vi "HardwareRead.vi"(8 "Error In":errorcluster, 10 "Setup":T2={"DUT"={"Count"=1, "Wirings"=[], "Names"=[]}, "Log"={"Start"={"Trigger Type"=enum."Immediate", "Timer (sec)"=0.0, "Digital IO Line"=0, "Digital IO Edge"=enum."Rising"}, "Rollover"={"Trigger Type"=enum."None", "Timer (sec)"=0.0, "File Size (MB)"=0, "Digital IO Line"=0, "Digital IO Edge"=enum."Rising"}, "Stop"={"Trigger Type"=enum."None", "Timer (sec)"=0.0, "File Size (MB)"=0, "Digital IO Line"=0, "Digital IO Edge"=enum."Rising"}}, "Trigger"={"Input"={"Type"=enum."None", "Timeout (ms)"=0, "Delay (ms)"=0, "Digital IO Line (1-14)"=0, "Digital IO Mode"=enum."Falling"}, "Output"={"Type"=enum."None", "Delay (ms)"=0, "Digital IO Line (1-14)"=0, "Digital IO Mode"=enum."Falling", "Digital IO Pulse Width (sec)"=0.0}}, "Sources"=[], "Measures"=[]} {"Measures"."Count" min=1 step=1; "Trigger"."Output"."Digital IO Line (1-14)" min=1 max=14 step=1}, 11 "Keithley 2602 In":refnum<visa-resource-name>) -> (0 "Error Out":errorcluster, 2 "Hardware Display Data":T1, 3 "Keithley 2602 Out":refnum<visa-resource-name>)   [LabVIEW 2013]
uses:
  Setup.ctl
  DUTConfiguration.ctl
  driver/Public/Controls/SMUSense.ctl
  LogConfiguration.ctl
  LogStartConfiguration.ctl
  LogStartTriggerType.ctl
  LogDigitalIOTriggerEdge.ctl
  LogRolloverConfiguration.ctl
  LogRolloverTriggerType.ctl
  LogStopConfiguration.ctl
  LogStopTriggerType.ctl
  TriggerConfiguration.ctl
  TriggerInputConfiguration.ctl
  TriggerInputType.ctl
  driver/Public/Controls/TriggerMode.ctl
  TriggerOutputConfiguration.ctl
  TriggerOutputType.ctl
  SourceConfiguration.ctl
  SourceFunction.ctl
  MeasureConfiguration.ctl
  HardwareDisplayData.ctl
  HardwareAbortGlobalAction.ctl
  driver/Keithley-2602.lvlib
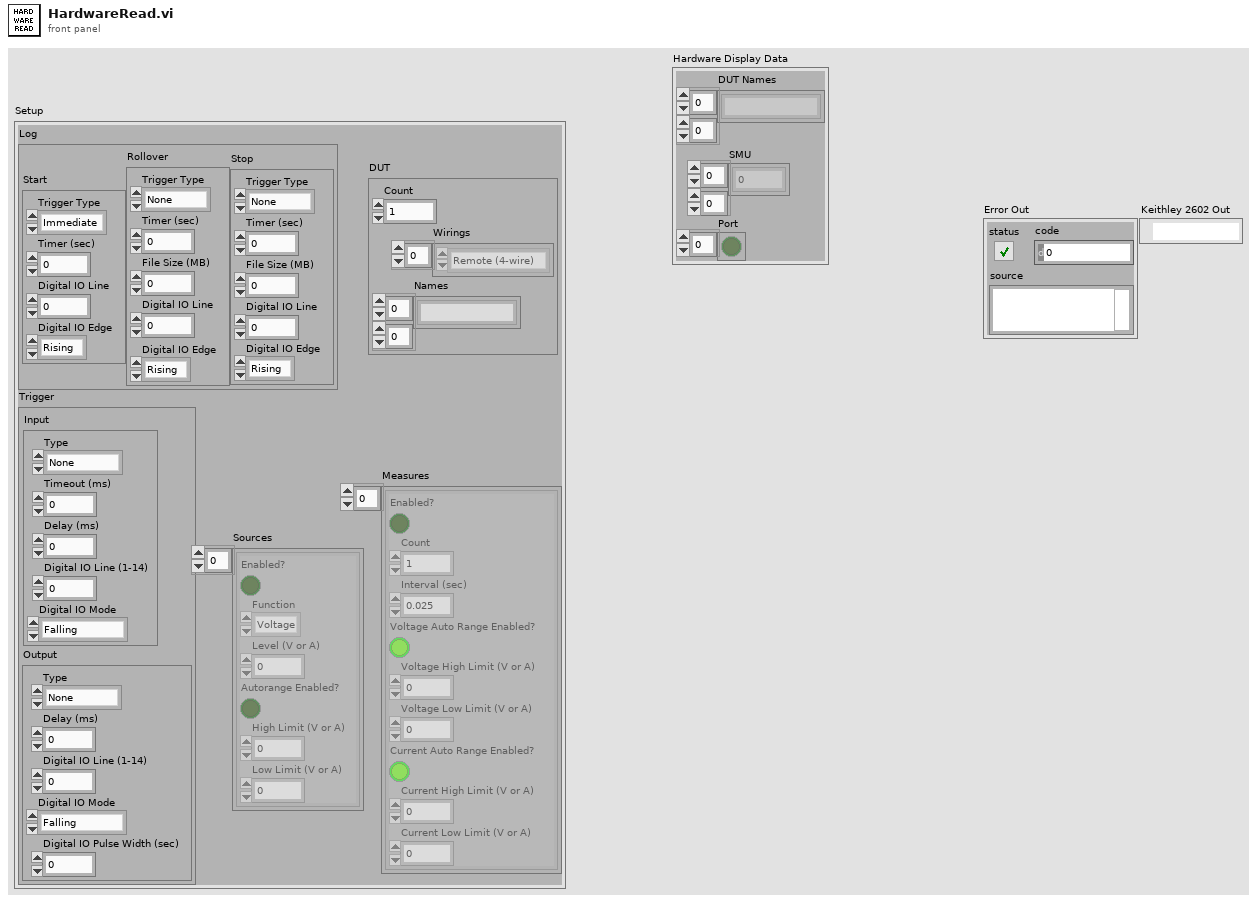
[diagram p1: front panel]
types:
  T1 = typedef "HardwareDisplayData.ctl" = cluster{"DUT Names":string[][], "SMU":dbl[][], "Port":bool[]}
  T2 = typedef "Setup.ctl" = cluster{"DUT":T3, "Log":T5, "Trigger":T13, "Sources":T19[], "Measures":T21[]}
  T3 = typedef "DUTConfiguration.ctl" = cluster{"Count":u32, "Wirings":T4[], "Names":string[][]}
  T4 = typedef "Keithley-2602.lvlib/SMUSense.ctl" = enum16{"Local (2-wire)", "Remote (4-wire)", "Calibration"}
  T5 = typedef "LogConfiguration.ctl" = cluster{"Start":T6, "Rollover":T9, "Stop":T11}
  T6 = typedef "LogStartConfiguration.ctl" = cluster{"Trigger Type":T7, "Timer (sec)":dbl, "Digital IO Line":u8, "Digital IO Edge":T8}
  T7 = typedef "LogStartTriggerType.ctl" = enum16{"Immediate", "User", "Timer", "Digital IO"}
  T8 = typedef "LogDigitalIOTriggerEdge.ctl" = enum16{"Rising", "Falling"}
  T9 = typedef "LogRolloverConfiguration.ctl" = cluster{"Trigger Type":T10, "Timer (sec)":dbl, "File Size (MB)":u32, "Digital IO Line":u8, "Digital IO Edge":T8}
  T10 = typedef "LogRolloverTriggerType.ctl" = enum16{"None", "Timer", "File Size", "Digital IO"}
  T11 = typedef "LogStopConfiguration.ctl" = cluster{"Trigger Type":T12, "Timer (sec)":dbl, "File Size (MB)":u32, "Digital IO Line":u8, "Digital IO Edge":T8}
  T12 = typedef "LogStopTriggerType.ctl" = enum16{"None", "User", "Timer", "File Size", "Digital IO"}
  T13 = typedef "TriggerConfiguration.ctl" = cluster{"Input":T14, "Output":T17}
  T14 = typedef "TriggerInputConfiguration.ctl" = cluster{"Type":T15, "Timeout (ms)":u32, "Delay (ms)":u32, "Digital IO Line (1-14)":u8, "Digital IO Mode":T16}
  T15 = typedef "TriggerInputType.ctl" = enum16{"None", "Digital IO", "Bus"}
  T16 = typedef "Keithley-2602.lvlib/TriggerMode.ctl" = enum16{"Falling", "Rising", "Either", "Synchronous"}
  T17 = typedef "TriggerOutputConfiguration.ctl" = cluster{"Type":T18, "Delay (ms)":u32, "Digital IO Line (1-14)":u8, "Digital IO Mode":T16, "Digital IO Pulse Width (sec)":dbl}
  T18 = typedef "TriggerOutputType.ctl" = enum16{"None", "Digital IO", "Bus"}
  T19 = typedef "SourceConfiguration.ctl" = cluster{"Enabled?":bool, "Function":T20, "Level (V or A)":dbl, "Autorange Enabled?":bool, "High Limit (V or A)":dbl, "Low Limit (V or A)":dbl}
  T20 = typedef "SourceFunction.ctl" = enum16{"Voltage", "Current"}
  T21 = typedef "MeasureConfiguration.ctl" = cluster{"Enabled?":bool, "Count":u8, "Interval (sec)":dbl, "Voltage Auto Range Enabled?":bool, "Voltage High Limit (V or A)":dbl, "Voltage Low Limit (V or A)":dbl, "Current Auto Range Enabled?":bool, "Current High Limit (V or A)":dbl, "Current Low Limit (V or A)":dbl}
  T22 = typedef "HardwareAbortGlobalAction.ctl" = enum16{"Set", "Get"}
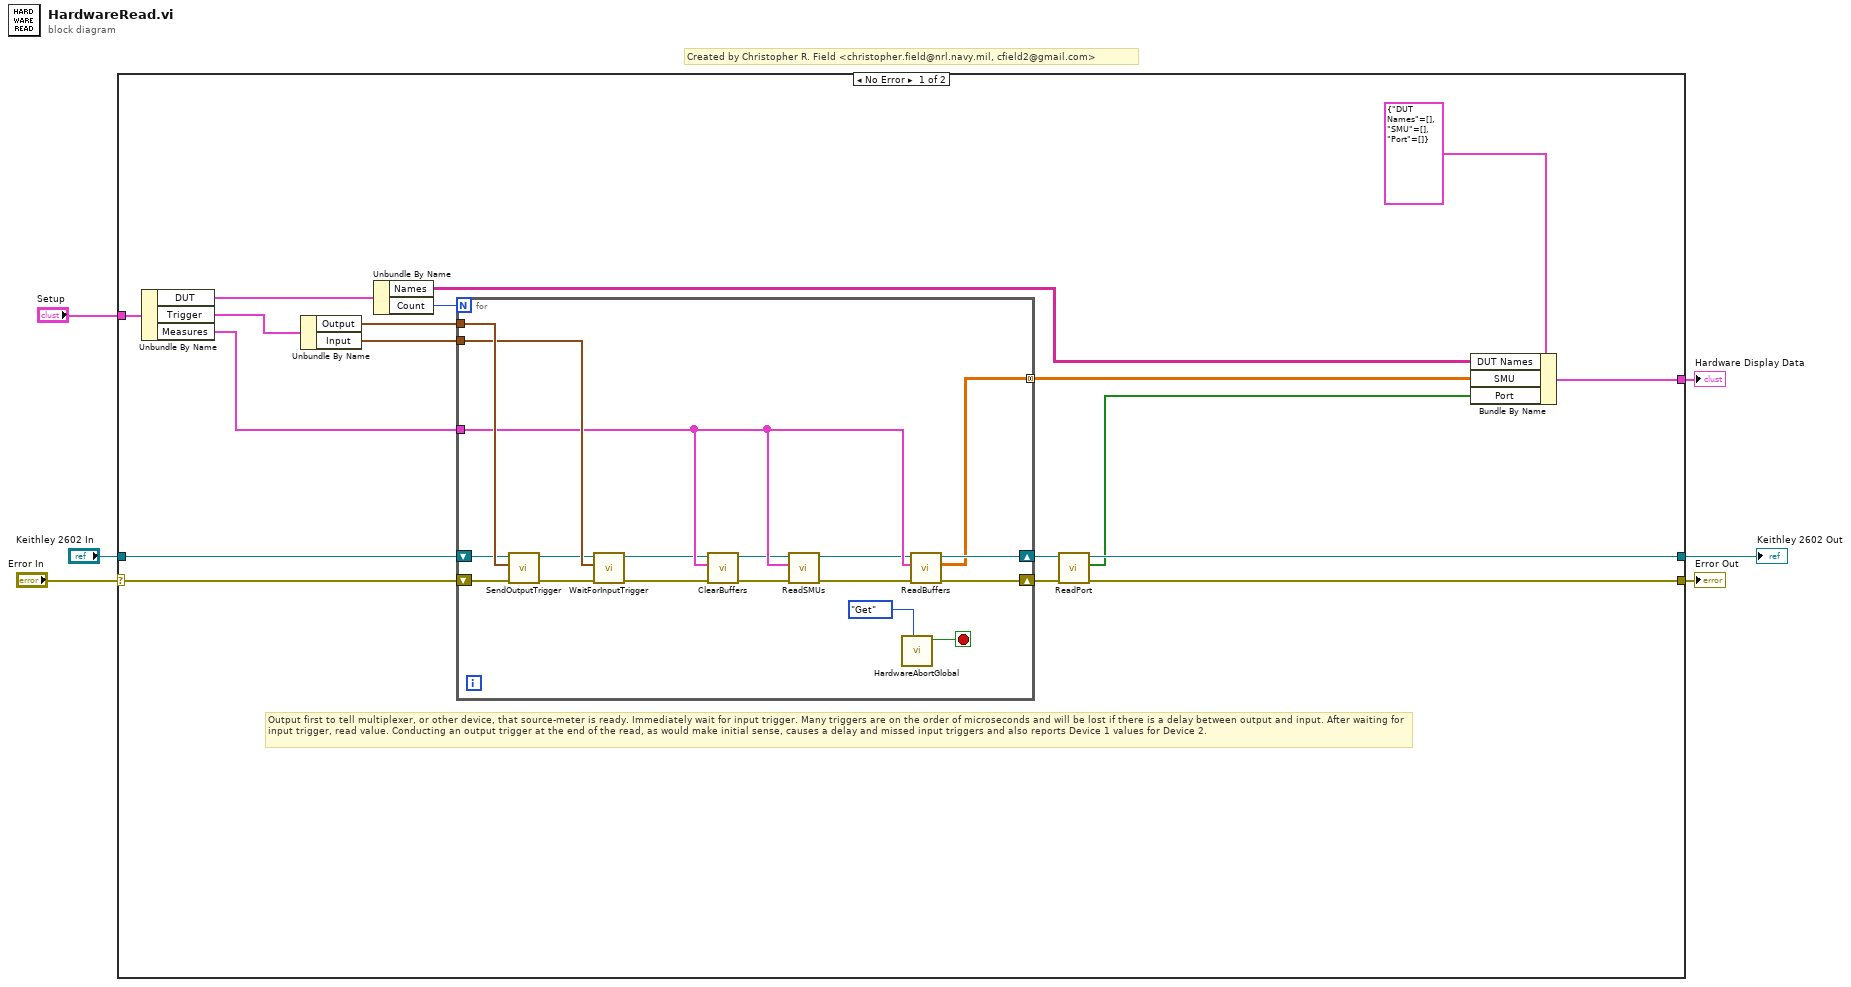
[diagram p0: block diagram]
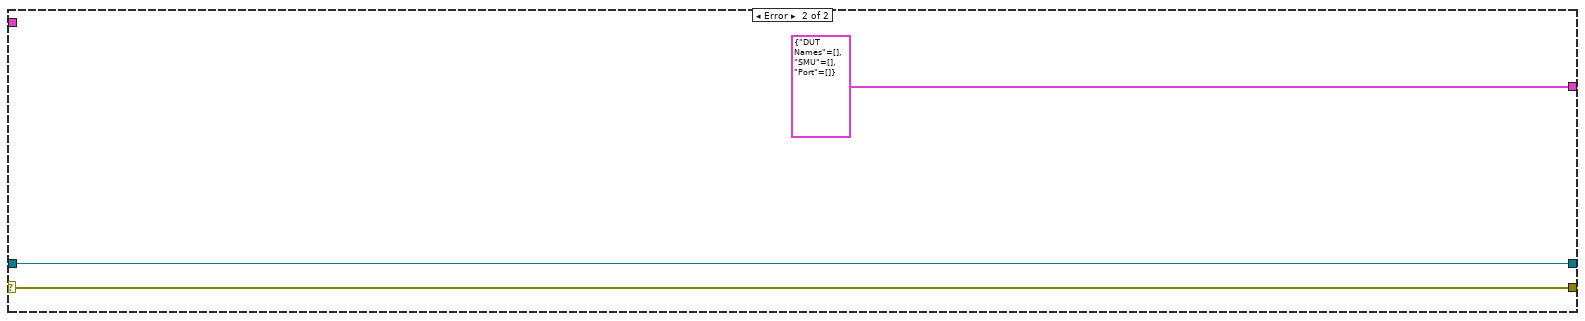
[diagram p2: hidden frame]
diagram:
  # "Created by Christopher R. Field <christopher.field@nrl.navy.mil, cfield2@gmail.com>"
  n1 = case shown="No Error" "Error In" {
    selector: "Error In" -> [w7 w44]
    tunnel: "Keithley 2602 In" -> [w8 w45]
    tunnel: [w18 w44] -> w4
    tunnel: [w19 w45] -> w3
    tunnel: "Setup" -> [w24 _]
    tunnel: [w10 T1 {"DUT Names"=[], "SMU"=[], "Port"=[]} ("Hardware Display Data")] -> w1
    frame No Error {
      # "Output first to tell multiplexer, or other device, that source-meter is ready. Immediately wait for input trigger. Many triggers are on the order of microseconds and will be lost if there is a delay between output and input. After waiting for input trigger, read value. Conducting an output trigger at the end of the read, as would make initial sense, causes a delay and missed input triggers and also reports Device 1 values for Device 2."
      n2 = Unbundle By Name(w24) -> ("DUT"=w15:T3, "Trigger"=w22:T13, "Measures"=w16:T21[])
      n3 = Unbundle By Name(w22) -> ("Output"=w9:T17, "Input"=w23:T14)
      n4 = Unbundle By Name(w15) -> ("Names"=w11:string[][], "Count"=w17:u32)
      n5 = for {
        N: w17 -> [_]
        shift-right: [w40] -> w20
        shift-left: w7 -> [w33]
        tunnel: w9 -> [w42]
        tunnel: w23 -> [w41]
        tunnel: [w38] -> w12 mode=concatenating
        tunnel: w16 -> [w35]
        shift-right: [w39] -> w21
        shift-left: w8 -> [w34]
        stop <- w36 stop-if-true
        n6 = call "SendOutputTrigger.vi"("Error In"=w33, "Output Trigger Configuration"=w42, "Keithley 2602 In"=w34) -> ("Error Out"=w31:errorcluster, "Keithley 2602 Out"=w32:refnum<visa-resource-name>)  [unwired: 7 in]
        n7 = call "WaitForInputTrigger.vi"("Error In"=w31, "Trigger Input Configuration"=w41, "Kiethley 2602 In"=w32) -> ("Error Out"=w30:errorcluster, "Keithley 2602 Out"=w29:refnum<visa-resource-name>)  [unwired: 7 in]
        n8 = call "ClearBuffers.vi"("Error In"=w30, "Measure Configurations"=w35, "Keithley 2602 In"=w29) -> ("Error Out"=w25:errorcluster, "Keithley 2602 Out"=w28:refnum<visa-resource-name>)  [unwired: 7 in]
        n9 = call "ReadSMUs.vi"("Error In"=w25, "Measure Configurations"=w35, "Keithley 2602 In"=w28) -> ("Error Out"=w26:errorcluster, "Keithley 2602 Out"=w27:refnum<visa-resource-name>)  [unwired: 7 in]
        n10 = call "HardwareAbortGlobal.vi"("Action"=HardwareAbortGlobalAction."Get") -> ("Value Out"=w36:bool)  [unwired: 10 in]
        n11 = call "ReadBuffers.vi"("Error In"=w26, "Measure Configurations"=w35, "Kiethley 2602 In"=w27) -> ("Error Out"=w40:errorcluster, "Data"=w38:dbl[][], "Keithley 2602 Out"=w39:refnum<visa-resource-name>)  [unwired: 6 in]
      }
      n12 = call "ReadPort.vi"("Error In"=w20, "Kiethley 2602 In"=w21) -> ("Error Out"=w18:errorcluster, "Port"=w13:bool[], "Keithley 2602 Out"=w19:refnum<visa-resource-name>)  [unwired: 7 in]
      n13 = Bundle By Name(cluster=T1 {"DUT Names"=[], "SMU"=[], "Port"=[]} ("Hardware Display Data"), "DUT Names"=w11, "SMU"=w12, "Port"=w13) -> (w10:T1)
    }
    frame Error {
    }
  }
  "Error Out" <- w4
  "Keithley 2602 Out" <- w3
  "Hardware Display Data" <- w1
